vi "HEWH Channel Test Labels.vi"() -> (6 "Chanel List":string, 8 "Label List":string[](array[string]), 10 "Pannel List":string[](array[string]))   [LabVIEW 2012]
uses:
  Channel Label.ctl
  <vilib>/Utility/file.llb/Write To Spreadsheet File (string).vi
  <vilib>/Utility/file.llb/Read From Spreadsheet File (string).vi
panel:
  in  "Read":bool
  in  "Write":bool
  in  "Sensor 4":T1
  in  "Read None":bool
  in  "Sensor 3":T1
  in  "Read All":bool
  in  "Initialize":bool
  in  "Complete":bool
  in  "Panel 3":T1[][](array[typedef])=[[{"Label"="TC Cond1 - IN", "Chan"="301", "Rec"=TRUE}, {"Label"="TC Cond2", "Chan"="302", "Rec"=TRUE}, {"Label"="TC Cond3", "Chan"="303", "Rec"=TRUE}, {"Label"="TC Cond4", "Chan"="304", "Rec"=TRUE}, {"Label"="TC Cond5", "Chan"="305", "Rec"=TRUE}, {"Label"="TC Cond6", "Chan"="306", "Rec"=TRUE}], [{"Label"="TC Cond7", "Chan"="307", "Rec"=TRUE}, {"Label"="TC Cond8", "Chan"="308", "Rec"=TRUE}, {"Label"="TC Cond9", "Chan"="309", "Rec"=TRUE}, {"Label"="TC Cond10", "Chan"="310", "Rec"=TRUE}, {"Label"="TC Cond11", "Chan"="311", "Rec"=TRUE}, {"Label"="TC Cond12 - OUT", "Chan"="312", "Rec"=TRUE}], [{"Label"="TC Xtra 4", "Chan"="313", "Rec"=TRUE}, {"Label"="TC Xtra 5", "Chan"="314", "Rec"=TRUE}, {"Label"="TC Xtra 6", "Chan"="315", "Rec"=TRUE}, {"Label"="TC Xtra 7", "Chan"="316", "Rec"=TRUE}, {"Label"="TC Xtra 8", "Chan"="105", "Rec"=TRUE}, {"Label"="TC Xtra 9", "Chan"="106", "Rec"=TRUE}]]
  in  "Panel 2":T1[][](array[typedef])=[[{"Label"="TC Dry/W bulb 1", "Chan"="201", "Rec"=TRUE}, {"Label"="TC Dry/W bulb 2", "Chan"="202", "Rec"=TRUE}, {"Label"="TC Dry/W bulb 3", "Chan"="203", "Rec"=TRUE}, {"Label"="TC Dry/W bulb 4", "Chan"="204", "Rec"=TRUE}, {"Label"="TC Tsuction", "Chan"="205", "Rec"=TRUE}, {"Label"="TC Tdis", "Chan"="206", "Rec"=TRUE}], [{"Label"="TC Tret", "Chan"="207", "Rec"=TRUE}, {"Label"="TC Controls 1", "Chan"="208", "Rec"=TRUE}, {"Label"="TC Controls 2", "Chan"="209", "Rec"=TRUE}, {"Label"="TC Controls 3", "Chan"="210", "Rec"=TRUE}, {"Label"="TC Controls 4", "Chan"="211", "Rec"=TRUE}, {"Label"="TC Controls 5", "Chan"="212", "Rec"=TRUE}], [{"Label"="TC Shadow T1", "Chan"="213", "Rec"=TRUE}, {"Label"="TC Shadow T2", "Chan"="214", "Rec"=TRUE}, {"Label"="TC Shadow T3", "Chan"="215", "Rec"=TRUE}, {"Label"="TC Shadow T4", "Chan"="216", "Rec"=TRUE}, {"Label"="TC Shadow T5", "Chan"="107", "Rec"=TRUE}, {"Label"="TC Shadow T6", "Chan"="108", "Rec"=TRUE}]]
  in  "Panel 1":T1[][](array[typedef])=[[{"Label"="TC Tree 1 - TOP", "Chan"="", "Rec"=TRUE}, {"Label"="TC Tree 2", "Chan"="", "Rec"=TRUE}, {"Label"="TC Tree 3", "Chan"="", "Rec"=TRUE}, {"Label"="TC Tree 4", "Chan"="", "Rec"=TRUE}, {"Label"="TC Tree 5", "Chan"="", "Rec"=TRUE}, {"Label"="TC Tree 6 - BOT", "Chan"="", "Rec"=TRUE}], [{"Label"="TC Shell 1", "Chan"="", "Rec"=TRUE}, {"Label"="TC Shell 2", "Chan"="", "Rec"=TRUE}, {"Label"="TC Shell 3", "Chan"="", "Rec"=TRUE}, {"Label"="TC Shell 4", "Chan"="", "Rec"=TRUE}, {"Label"="TC Evap1 - IN", "Chan"="111", "Rec"=TRUE}, {"Label"="TC Evap2", "Chan"="112", "Rec"=TRUE}], [{"Label"="TC Evap3", "Chan"="113", "Rec"=TRUE}, {"Label"="TC Evap4", "Chan"="114", "Rec"=TRUE}, {"Label"="TC Evap5 - OUT", "Chan"="115", "Rec"=TRUE}, {"Label"="TC Xtra 1", "Chan"="116", "Rec"=TRUE}, {"Label"="TC Xtra 2", "Chan"="109", "Rec"=TRUE}, {"Label"="TC Xtra 3", "Chan"="1100", "Rec"=TRUE}]]
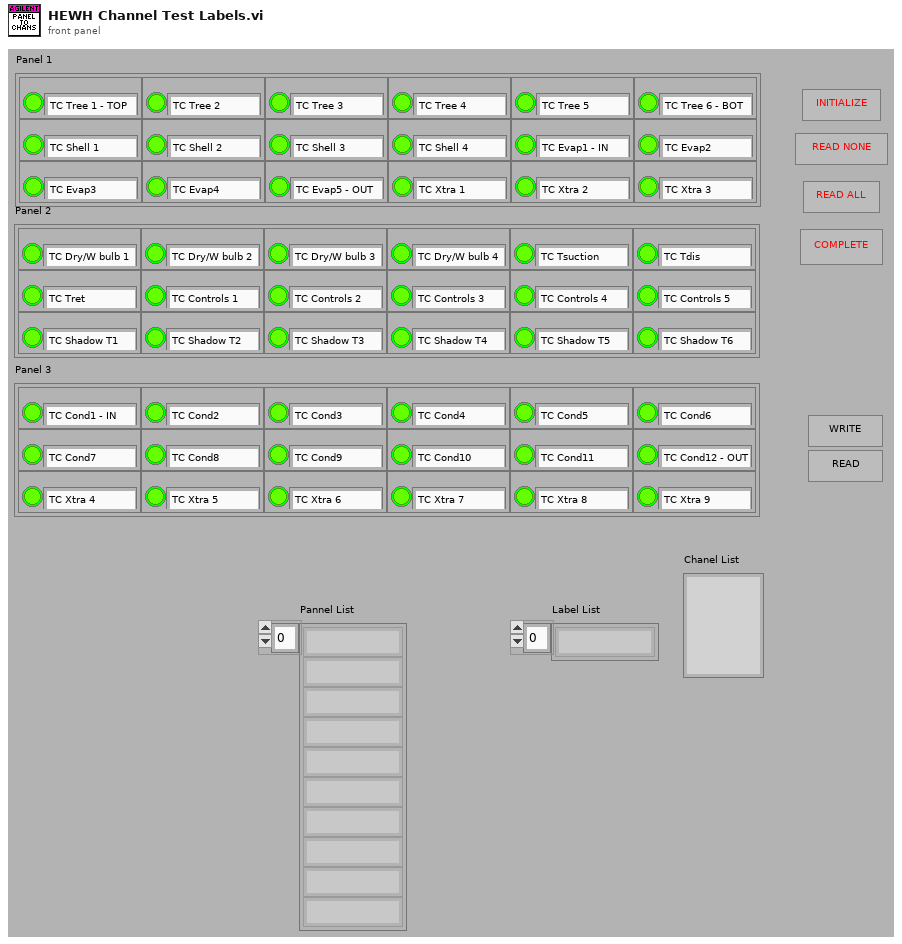
[diagram p1: front panel]
types:
  T1 = typedef "Channel Label.ctl" = cluster{"Label":string, "Chan":string, "Rec":bool}
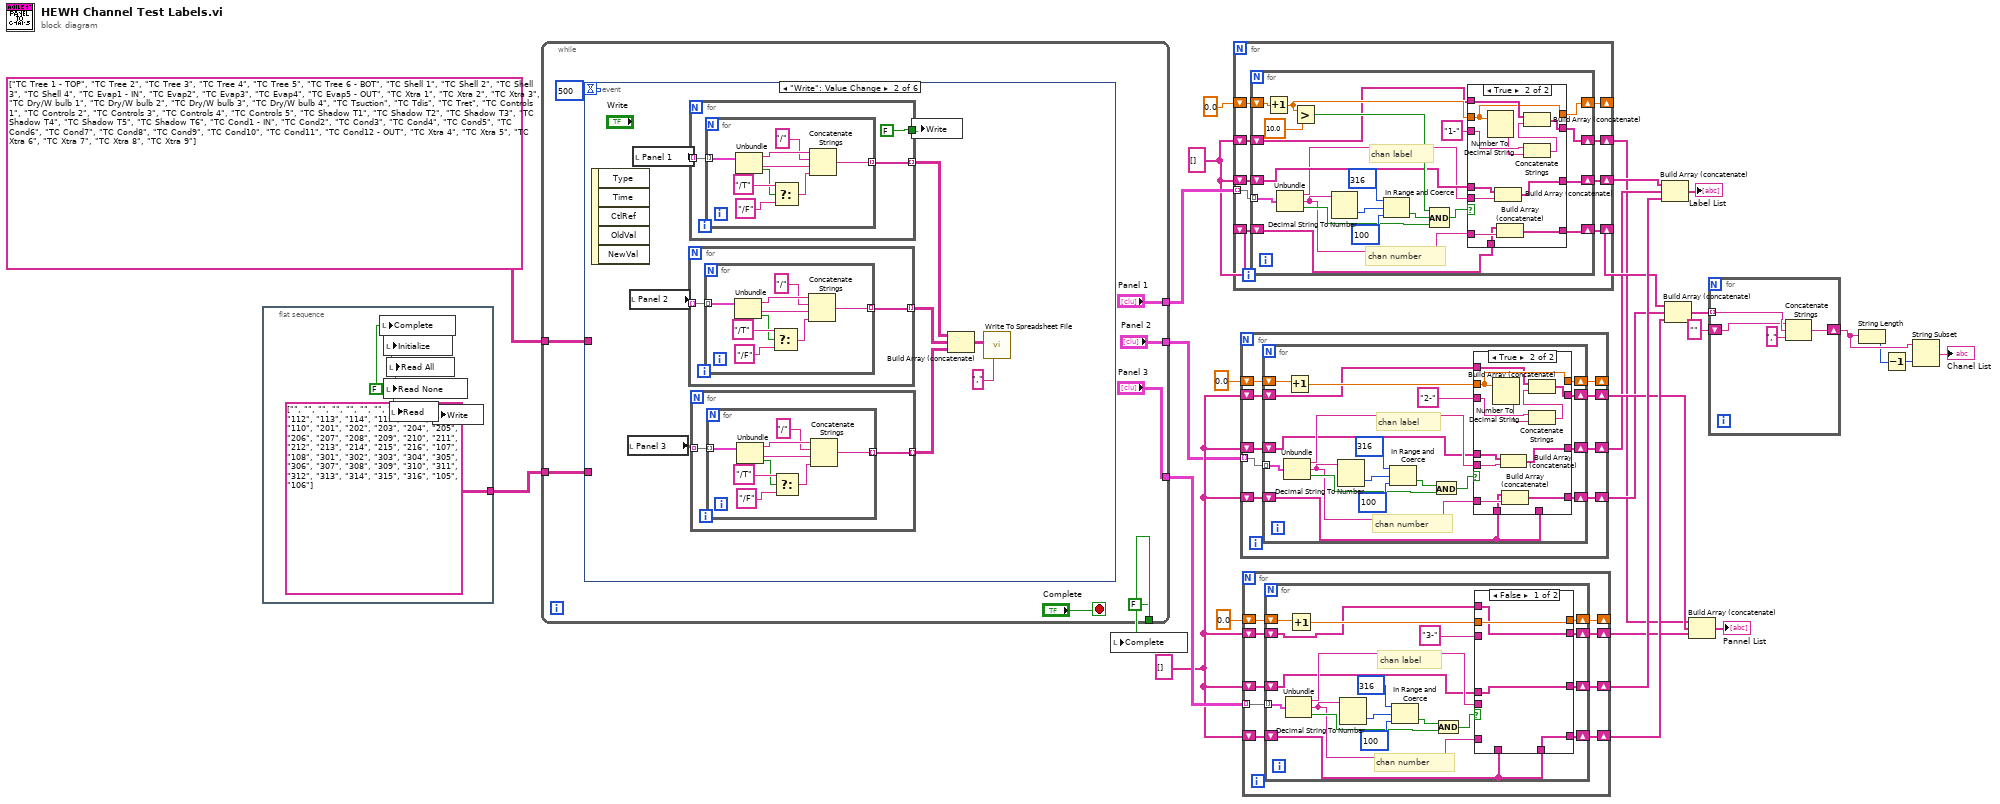
[diagram p0: block diagram]
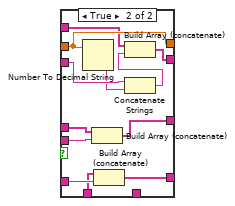
[diagram p3: hidden frame]
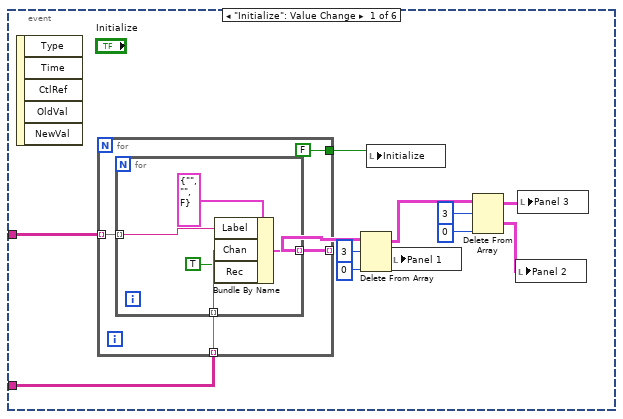
[diagram p5: hidden frame]
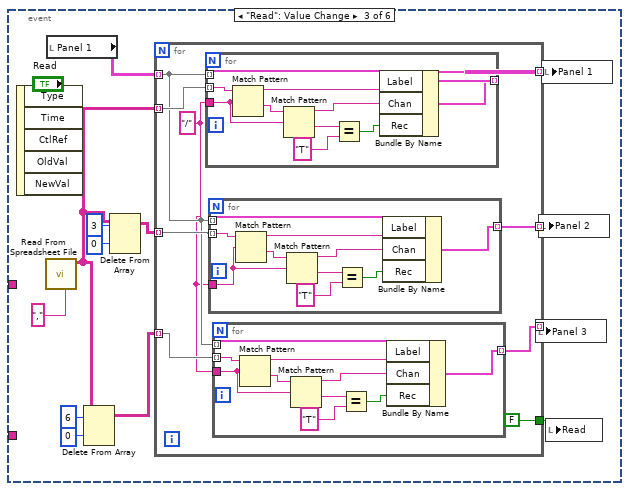
[diagram p6: hidden frame]
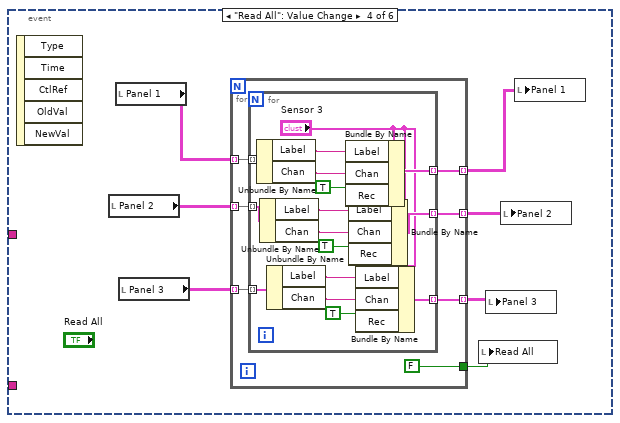
[diagram p7: hidden frame]
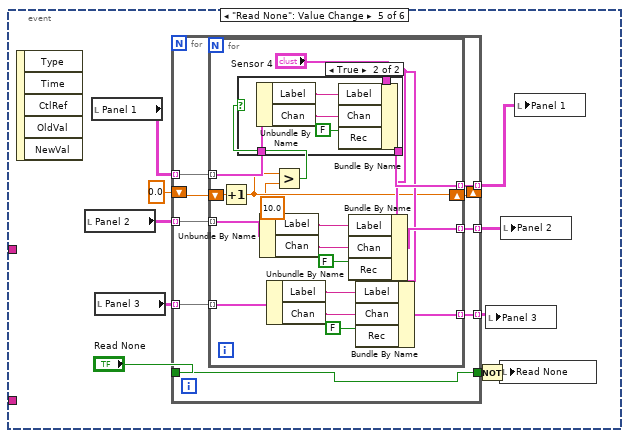
[diagram p8: hidden frame]
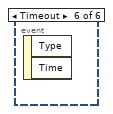
[diagram p10: hidden frame]
diagram:
  w6 = string[] []
  w2 = string[] []
  n1 = flat-sequence {
    tunnel: [string[][] [["", "", "", "", "", ""], ["", "", "", "", "111", "112"], ["113", "114", "115", "116", "109", "110"], ["201", "202", "203", "204", "205", "206"], ["207", "208", "209", "210", "211", "212"], ["213", "214", "215", "216", "107", "108"], ["301", "302", "303", "304", "305", "306"], ["307", "308", "309", "310", "311", "312"], ["313", "314", "315", "316", "105", "106"]] ("transposed array")] -> w27
    frame #0 {
      w29 = FALSE ("Read None")
      n2 = local write "Complete"(w29) -> ()
      n3 = local write "Initialize"(w29) -> ()
      n4 = local write "Read None"(w29) -> ()
      n5 = local write "Read All"(w29) -> ()
      n6 = local write "Read"(w29) -> ()
      n7 = local write "Write"(w29) -> ()
    }
  }
  n8 = while {
    tunnel: string[][] [["TC Tree 1 - TOP", "TC Tree 2", "TC Tree 3", "TC Tree 4", "TC Tree 5", "TC Tree 6 - BOT"], ["TC Shell 1", "TC Shell 2", "TC Shell 3", "TC Shell 4", "TC Evap1 - IN", "TC Evap2"], ["TC Evap3", "TC Evap4", "TC Evap5 - OUT", "TC Xtra 1", "TC Xtra 2", "TC Xtra 3"], ["TC Dry/W bulb 1", "TC Dry/W bulb 2", "TC Dry/W bulb 3", "TC Dry/W bulb 4", "TC Tsuction", "TC Tdis"], ["TC Tret", "TC Controls 1", "TC Controls 2", "TC Controls 3", "TC Controls 4", "TC Controls 5"], ["TC Shadow T1", "TC Shadow T2", "TC Shadow T3", "TC Shadow T4", "TC Shadow T5", "TC Shadow T6"], ["TC Cond1 - IN", "TC Cond2", "TC Cond3", "TC Cond4", "TC Cond5", "TC Cond6"], ["TC Cond7", "TC Cond8", "TC Cond9", "TC Cond10", "TC Cond11", "TC Cond12 - OUT"], ["TC Xtra 4", "TC Xtra 5", "TC Xtra 6", "TC Xtra 7", "TC Xtra 8", "TC Xtra 9"]] ("Array") -> [w38]
    tunnel: w27 -> [w37]
    tunnel: ["Panel 1"] -> w26
    tunnel: ["Panel 2"] -> w5
    tunnel: ["Panel 3"] -> w25
    tunnel: [FALSE ("Read None")] -> w19
    stop <- "Complete" stop-if-true
    n9 = event shown="[1] \"Write\": Value Change" {
      selector: _ -> [_ _ _ _ _ _]
      dyn-events: _ -> [_ _ _ _ _ _]
      timeout: 500 -> [_ _ _ _ _ _]
      tunnel: w38 -> [w50 _ _ _ _ _]
      tunnel: w37 -> [w49 _ _ _ _ _]
      event "Initialize": Value Change {
        n10 = event-data() -> ()  [unwired: 1 in, 5 out]
        n11 = for {
          tunnel: [w54] -> w48 mode=indexing
          tunnel: w50 -> [w53] mode=indexing
          tunnel: w49 -> [w52] mode=indexing
          tunnel: [FALSE ("Read None")] -> w39
          n12 = for {
            tunnel: [w59] -> w54 mode=indexing
            tunnel: w53 -> [w58] mode=indexing
            tunnel: w52 -> [w57] mode=indexing
            n13 = Bundle By Name(cluster=T1 {"Label"="", "Chan"="", "Rec"=FALSE} ("Sensor 2"), "Label"=w58, "Chan"=w57, "Rec"=TRUE) -> (w59:T1)
          }
        }
        n14 = Delete From Array(array=w48, length=3, index (row)=0) -> (deleted portion=w42:T1[][], array with subset deleted=w43:T1[][])  [unwired: 1 in]
        n15 = local write "Initialize"(w39) -> ()
        n16 = local write "Panel 1"(w42) -> ()
        n17 = Delete From Array(array=w43, length=3, index (row)=0) -> (deleted portion=w41:T1[][], array with subset deleted=w40:T1[][])  [unwired: 1 in]
        n18 = local write "Panel 2"(w41) -> ()
        n19 = local write "Panel 3"(w40) -> ()
      }
      event "Write": Value Change {
        n20 = event-data() -> ()  [unwired: 1 in, 5 out]
        n21 = local read "Panel 3"() -> (w64:T1[][])
        n22 = local read "Panel 2"() -> (w65:T1[][])
        n23 = local read "Panel 1"() -> (w67:T1[][])
        n24 = for {
          tunnel: w65 -> [w81] mode=indexing
          tunnel: [w80] -> w62 mode=indexing
          n25 = for {
            tunnel: w81 -> [w90] mode=indexing
            tunnel: [w82] -> w80 mode=indexing
            n26 = Unbundle(w90) -> ("Label"=w89:string, "Chan"=w87:string, "Rec"=w84:bool)
            n27 = Select(t="/T" ("string"), s=w84, f="/F" ("string")) -> (s? t:f=w83:string)
            n28 = Concatenate Strings(w89, "/" ("string"), w87, w83) -> (w82:string)
          }
        }
        n29 = for {
          tunnel: w67 -> [w93] mode=indexing
          tunnel: [FALSE ("Read None")] -> w68
          tunnel: [w91] -> w63 mode=indexing
          n30 = for {
            tunnel: w93 -> [w102] mode=indexing
            tunnel: [w94] -> w91 mode=indexing
            n31 = Unbundle(w102) -> ("Label"=w101:string, "Chan"=w99:string, "Rec"=w96:bool)
            n32 = Select(t="/T" ("string"), s=w96, f="/F" ("string")) -> (s? t:f=w95:string)
            n33 = Concatenate Strings(w101, "/" ("string"), w99, w95) -> (w94:string)
          }
        }
        n34 = for {
          tunnel: w64 -> [w70] mode=indexing
          tunnel: [w69] -> w61 mode=indexing
          n35 = for {
            tunnel: w70 -> [w79] mode=indexing
            tunnel: [w71] -> w69 mode=indexing
            n36 = Unbundle(w79) -> ("Label"=w78:string, "Chan"=w76:string, "Rec"=w73:bool)
            n37 = Select(t="/T" ("string"), s=w73, f="/F" ("string")) -> (s? t:f=w72:string)
            n38 = Concatenate Strings(w78, "/" ("string"), w76, w72) -> (w71:string)
          }
        }
        n39 = local write "Write"(w68) -> ()
        n40 = Build Array (concatenate)(w63, w62, w61) -> (w60:string[][])
        n41 = call-poly <vilib>:"Write To Spreadsheet File.vi"("delimiter (\\t)"="," ("delimiter (\\t)"), "2D data"=w60) -> ()  [unwired: 6 in, 1 out]
      }
      event "Read": Value Change {
        n42 = event-data() -> ()  [unwired: 1 in, 5 out]
        n43 = call-poly <vilib>:"Read From Spreadsheet File.vi"("delimiter (\\t)"="," ("delimiter (\\t)")) -> ("all rows"=w109:string[][])  [unwired: 6 in, 4 out]
        n44 = local read "Panel 1"() -> (w105:T1[][])
        n45 = Delete From Array(array=w109, length=6, index (row)=0) -> (array with subset deleted=w111:string[][])  [unwired: 1 in, 1 out]
        n46 = Delete From Array(array=w109, length=3, index (row)=0) -> (array with subset deleted=w110:string[][])  [unwired: 1 in, 1 out]
        n47 = for {
          tunnel: w105 -> [w119] mode=indexing
          tunnel: w109 -> [w124] mode=indexing
          tunnel: [w123] -> w108 mode=indexing
          tunnel: w110 -> [w122] mode=indexing
          tunnel: w111 -> [w118] mode=indexing
          tunnel: [w121] -> w107 mode=indexing
          tunnel: [w120] -> w106 mode=indexing
          tunnel: [FALSE ("Read")] -> w104
          w117 = "/" ("regular expression")
          n48 = for {
            tunnel: w119 -> [w153] mode=indexing
            tunnel: w124 -> [w154] mode=indexing
            tunnel: [w151] -> w123 mode=indexing
            tunnel: w117 -> [w145]
            n49 = Match Pattern(string=w154, regular expression=w145) -> (before substring=w152:string, after substring=w150:string)  [unwired: 1 in, 2 out]
            n50 = Match Pattern(string=w150, regular expression=w145) -> (before substring=w149:string, after substring=w148:string)  [unwired: 1 in, 2 out]
            n51 = Equal?(x=w148, y="T") -> (x = y?=w146:bool)
            n52 = Bundle By Name(cluster=w153, "Label"=w152, "Chan"=w149, "Rec"=w146) -> (w151:T1)
          }
          n53 = for {
            tunnel: w119 -> [w143] mode=indexing
            tunnel: w122 -> [w144] mode=indexing
            tunnel: [w141] -> w121 mode=indexing
            tunnel: w117 -> [w135]
            n54 = Match Pattern(string=w144, regular expression=w135) -> (before substring=w142:string, after substring=w140:string)  [unwired: 1 in, 2 out]
            n55 = Match Pattern(string=w140, regular expression=w135) -> (before substring=w139:string, after substring=w138:string)  [unwired: 1 in, 2 out]
            n56 = Equal?(x=w138, y="T") -> (x = y?=w136:bool)
            n57 = Bundle By Name(cluster=w143, "Label"=w142, "Chan"=w139, "Rec"=w136) -> (w141:T1)
          }
          n58 = for {
            tunnel: w119 -> [w133] mode=indexing
            tunnel: w118 -> [w134] mode=indexing
            tunnel: [w131] -> w120 mode=indexing
            tunnel: w117 -> [w125]
            n59 = Match Pattern(string=w134, regular expression=w125) -> (before substring=w132:string, after substring=w130:string)  [unwired: 1 in, 2 out]
            n60 = Match Pattern(string=w130, regular expression=w125) -> (before substring=w129:string, after substring=w128:string)  [unwired: 1 in, 2 out]
            n61 = Equal?(x=w128, y="T") -> (x = y?=w126:bool)
            n62 = Bundle By Name(cluster=w133, "Label"=w132, "Chan"=w129, "Rec"=w126) -> (w131:T1)
          }
        }
        n63 = local write "Panel 3"(w106) -> ()
        n64 = local write "Panel 2"(w107) -> ()
        n65 = local write "Panel 1"(w108) -> ()
        n66 = local write "Read"(w104) -> ()
      }
      event "Read All": Value Change {
        n67 = event-data() -> ()  [unwired: 1 in, 5 out]
        n68 = local read "Panel 2"() -> (w158:T1[][])
        n69 = local read "Panel 1"() -> (w161:T1[][])
        n70 = local read "Panel 3"() -> (w157:T1[][])
        n71 = for {
          tunnel: [w168] -> w160 mode=indexing
          tunnel: w161 -> [w167] mode=indexing
          tunnel: [w166] -> w159 mode=indexing
          tunnel: w158 -> [w165] mode=indexing
          tunnel: w157 -> [w164] mode=indexing
          tunnel: [w163] -> w156 mode=indexing
          tunnel: [FALSE ("Read None")] -> w155
          n72 = for {
            tunnel: [w184] -> w168 mode=indexing
            tunnel: w167 -> [w182] mode=indexing
            tunnel: [w176] -> w166 mode=indexing
            tunnel: w165 -> [w175] mode=indexing
            tunnel: w164 -> [w171] mode=indexing
            tunnel: [w170] -> w163 mode=indexing
            n73 = Unbundle By Name(w182) -> ("Label"=w181:string, "Chan"=w180:string)
            n74 = Unbundle By Name(w175) -> ("Label"=w178:string, "Chan"=w179:string)
            n75 = Unbundle By Name(w171) -> ("Label"=w173:string, "Chan"=w172:string)
            n76 = Bundle By Name(cluster="Sensor 3", "Label"=w181, "Chan"=w180, "Rec"=TRUE) -> (w184:T1)
            n77 = Bundle By Name(cluster="Sensor 3", "Label"=w178, "Chan"=w179, "Rec"=TRUE) -> (w176:T1)
            n78 = Bundle By Name(cluster="Sensor 3", "Label"=w173, "Chan"=w172, "Rec"=TRUE) -> (w170:T1)
          }
        }
        n79 = local write "Read All"(w155) -> ()
        n80 = local write "Panel 3"(w156) -> ()
        n81 = local write "Panel 2"(w159) -> ()
        n82 = local write "Panel 1"(w160) -> ()
      }
      event "Read None": Value Change {
        n83 = event-data() -> ()  [unwired: 1 in, 5 out]
        n84 = local read "Panel 2"() -> (w191:T1[][])
        n85 = local read "Panel 1"() -> (w194:T1[][])
        n86 = local read "Panel 3"() -> (w190:T1[][])
        n87 = for {
          tunnel: [w203] -> w193 mode=indexing
          tunnel: w194 -> [w202] mode=indexing
          tunnel: [w201] -> w192 mode=indexing
          tunnel: w191 -> [w200] mode=indexing
          tunnel: w190 -> [w199] mode=indexing
          tunnel: [w198] -> w189 mode=indexing
          tunnel: [w197] -> w187
          tunnel: "Read None" -> [w197]
          shift-right: [w195] -> _
          shift-left: 0.0 -> [w196]
          n88 = for {
            tunnel: [w220] -> w203 mode=indexing
            tunnel: w202 -> [w219] mode=indexing
            tunnel: [w215] -> w201 mode=indexing
            tunnel: w200 -> [w214] mode=indexing
            tunnel: w199 -> [w210] mode=indexing
            tunnel: [w209] -> w198 mode=indexing
            shift-right: [w206] -> w195
            shift-left: w196 -> [w207]
            n89 = Increment(x=w207) -> (x+1=w206:dbl)
            n90 = Unbundle By Name(w214) -> ("Label"=w217:string, "Chan"=w218:string)
            n91 = Unbundle By Name(w210) -> ("Label"=w212:string, "Chan"=w211:string)
            n92 = Greater?(x=w206, y=10.0) -> (0:w204:bool)
            n93 = case shown="True" w204 {
              tunnel: [w221 w227] -> w220
              tunnel: w219 -> [w221 w225]
              tunnel: "Sensor 4" -> [_ w222]
              frame False {
              }
              frame True {
                n94 = Unbundle By Name(w225) -> ("Label"=w224:string, "Chan"=w223:string)
                n95 = Bundle By Name(cluster=w222, "Label"=w224, "Chan"=w223, "Rec"=FALSE) -> (w227:T1)
              }
            }
            n96 = Bundle By Name(cluster="Sensor 4", "Label"=w217, "Chan"=w218, "Rec"=FALSE) -> (w215:T1)
            n97 = Bundle By Name(cluster="Sensor 4", "Label"=w212, "Chan"=w211, "Rec"=FALSE) -> (w209:T1)
          }
        }
        n98 = Not(x=w187) -> (.not. x?=w188:bool)
        n99 = local write "Panel 3"(w189) -> ()
        n100 = local write "Read None"(w188) -> ()
        n101 = local write "Panel 2"(w192) -> ()
        n102 = local write "Panel 1"(w193) -> ()
      }
      event Timeout {
        n103 = event-data() -> ()  [unwired: 1 in, 2 out]
      }
    }
  }
  n104 = local write "Complete"(w19) -> ()
  n105 = for {
    tunnel: w26 -> [w236] mode=indexing
    shift-right: [w235] -> w24
    shift-left: w2 -> [w234]
    shift-right: [w233] -> w20
    shift-left: w2 -> [w232]
    shift-right: [w230] -> _
    shift-left: 0.0 -> [w231]
    shift-right: [w228] -> w1
    shift-left: w2 -> [w229]
    n106 = for {
      tunnel: w236 -> [w257] mode=indexing
      shift-right: [w248] -> w235
      shift-left: w234 -> [w242]
      shift-right: [w238] -> w233
      shift-left: w232 -> [w239]
      shift-right: [w247] -> w230
      shift-left: w231 -> [w251]
      shift-right: [w244] -> w228
      shift-left: w229 -> [w245]
      # "chan label"
      # "chan number"
      n107 = Increment(x=w251) -> (x+1=w246:dbl)
      n108 = Unbundle(w257) -> ("Label"=w241:string, "Chan"=w240:string, "Rec"=w252:bool)
      n109 = Greater?(x=w246, y=10.0) -> (0:w249:bool)
      n110 = Decimal String To Number(string=w240) -> (number=w256:i32)  [unwired: 2 in, 1 out]
      n111 = In Range and Coerce(upper limit=316, x=w256, lower limit=100) -> (In Range?=w253:bool)  [unwired: 1 out]
      n112 = Compound Arithmetic op=AND(w249, w253, w252) -> (w243:bool)
      n113 = case shown="True" w243 {
        tunnel: w241 -> [_ w273]
        tunnel: [w261 w272] -> w248
        tunnel: w242 -> [w261 w270]
        tunnel: [w258 w271] -> w238
        tunnel: w240 -> [_ w269]
        tunnel: w239 -> [w258 w268]
        tunnel: w246 -> [w260 w262]
        tunnel: [w259 w267] -> w244
        tunnel: [w260 w262] -> w247
        tunnel: "1-" -> [_ w266]
        tunnel: w245 -> [w259 w263]
        frame False {
        }
        frame True {
          n114 = Number To Decimal String(number=w262) -> (decimal integer string=w265:string)  [unwired: 1 in]
          n115 = Build Array (concatenate)(w270, w273) -> (w272:string[])
          n116 = Build Array (concatenate)(w268, w269) -> (w271:string[])
          n117 = Concatenate Strings(w266, w265) -> (w264:string)
          n118 = Build Array (concatenate)(w263, w264) -> (w267:string[])
        }
      }
    }
  }
  n119 = for {
    tunnel: w5 -> [w282] mode=indexing
    shift-right: [w281] -> w3
    shift-left: w6 -> [w280]
    shift-right: [w279] -> w4
    shift-left: w6 -> [w278]
    shift-right: [w275] -> _
    shift-left: 0.0 -> [w277]
    shift-right: [w276] -> w7
    shift-left: w6 -> [w274]
    n120 = for {
      tunnel: w282 -> [w301] mode=indexing
      shift-right: [w294] -> w281
      shift-left: w280 -> [w293]
      shift-right: [w291] -> w279
      shift-left: w278 -> [w289]
      shift-right: [w285] -> w275
      shift-left: w277 -> [w288]
      shift-right: [w286] -> w276
      shift-left: w274 -> [w283]
      # "chan label"
      # "chan number"
      n121 = Unbundle(w301) -> ("Label"=w295:string, "Chan"=w290:string, "Rec"=w296:bool)
      n122 = Increment(x=w288) -> (x+1=w287:dbl)
      n123 = Decimal String To Number(string=w290) -> (number=w300:i32)  [unwired: 2 in, 1 out]
      n124 = In Range and Coerce(upper limit=316, x=w300, lower limit=100) -> (In Range?=w297:bool)  [unwired: 1 out]
      n125 = And(x=w297, y=w296) -> (x .and. y?=w292:bool)
      n126 = case shown="True" w292 {
        tunnel: w295 -> [_ w317]
        tunnel: [w305 w316] -> w294
        tunnel: w293 -> [w305 w314]
        tunnel: [w304 w315] -> w291
        tunnel: w290 -> [_ w313]
        tunnel: w289 -> [w304 _]
        tunnel: w289 -> [_ w312]
        tunnel: w287 -> [w303 w310]
        tunnel: [w302 w311] -> w286
        tunnel: [w303 w310] -> w285
        tunnel: "2-" -> [_ w309]
        tunnel: w283 -> [w302 w306]
        frame False {
        }
        frame True {
          n127 = Number To Decimal String(number=w310) -> (decimal integer string=w308:string)  [unwired: 1 in]
          n128 = Build Array (concatenate)(w314, w317) -> (w316:string[])
          n129 = Build Array (concatenate)(w312, w313) -> (w315:string[])
          n130 = Concatenate Strings(w309, w308) -> (w307:string)
          n131 = Build Array (concatenate)(w306, w307) -> (w311:string[])
        }
      }
    }
  }
  n132 = for {
    tunnel: w25 -> [w326] mode=indexing
    shift-right: [w325] -> w23
    shift-left: w6 -> [w324]
    shift-right: [w323] -> w21
    shift-left: w6 -> [w322]
    shift-right: [w319] -> _
    shift-left: 0.0 -> [w321]
    shift-right: [w320] -> w9
    shift-left: w6 -> [w318]
    n133 = for {
      tunnel: w326 -> [w345] mode=indexing
      shift-right: [w338] -> w325
      shift-left: w324 -> [w337]
      shift-right: [w335] -> w323
      shift-left: w322 -> [w333]
      shift-right: [w329] -> w319
      shift-left: w321 -> [w332]
      shift-right: [w330] -> w320
      shift-left: w318 -> [w327]
      # "chan label"
      # "chan number"
      n134 = Unbundle(w345) -> ("Label"=w339:string, "Chan"=w334:string, "Rec"=w340:bool)
      n135 = Increment(x=w332) -> (x+1=w331:dbl)
      n136 = Decimal String To Number(string=w334) -> (number=w344:i32)  [unwired: 2 in, 1 out]
      n137 = In Range and Coerce(upper limit=316, x=w344, lower limit=100) -> (In Range?=w341:bool)  [unwired: 1 out]
      n138 = And(x=w341, y=w340) -> (x .and. y?=w336:bool)
      n139 = case shown="False" w336 {
        tunnel: w339 -> [_ w361]
        tunnel: [w349 w360] -> w338
        tunnel: w337 -> [w349 w358]
        tunnel: [w348 w359] -> w335
        tunnel: w334 -> [_ w357]
        tunnel: w333 -> [w348 _]
        tunnel: w333 -> [_ w356]
        tunnel: w331 -> [w347 w354]
        tunnel: [w346 w355] -> w330
        tunnel: [w347 w354] -> w329
        tunnel: "3-" -> [_ w353]
        tunnel: w327 -> [w346 w350]
        frame False {
        }
        frame True {
          n140 = Number To Decimal String(number=w354) -> (decimal integer string=w352:string)  [unwired: 1 in]
          n141 = Build Array (concatenate)(w358, w361) -> (w360:string[])
          n142 = Build Array (concatenate)(w356, w357) -> (w359:string[])
          n143 = Concatenate Strings(w353, w352) -> (w351:string)
          n144 = Build Array (concatenate)(w350, w351) -> (w355:string[])
        }
      }
    }
  }
  n145 = Build Array (concatenate)(w24, w3, w23) -> (→"Label List":string[])
  n146 = Build Array (concatenate)(w20, w4, w21) -> (w18:string[])
  n147 = Build Array (concatenate)(w1, w7, w9) -> (→"Pannel List":string[])
  n148 = for {
    tunnel: w18 -> [w364] mode=indexing
    shift-right: [w363] -> w16
    shift-left: "" -> [w362]
    n149 = Concatenate Strings(w362, w364, "," ("string")) -> (w363:string)
  }
  n150 = String Length(string=w16) -> (length=w14:i32)
  n151 = Decrement(x=w14) -> (x-1=w15:i32)
  n152 = String Subset(string=w16, length (rest)=w15) -> (substring=→"Chanel List":string)  [unwired: 1 in]
